vi "Initialize Central Message Handler.vi"(8 "Error In":errorcluster, 11 "Dashboard In":refnum<class "Dashboard.lvclass">) -> (0 "Error Out":errorcluster, 3 "Dashboard Out":refnum<class "Dashboard.lvclass">)   [LabVIEW 2019, in "Dashboard.lvclass"]
uses:
  Dashboard.lvclass
  Accessors/Processes/Get Processes.vi
  Process/Accessors/Message Queue/Get Message Queue.vi
  Accessors/Central Message Handler/Set Central Message Handler.vi
  Display Manager/Display Manager.lvclass
  Audio Analyzer/Audio Analyzer.lvclass
  Draw Frame/Draw Frame.lvclass
  Error Handling/Error Handling.lvclass
  Sequencer/Sequencer.lvclass
  Central Message Handler/Central Message Handler.lvclass
  Process/Process.lvclass
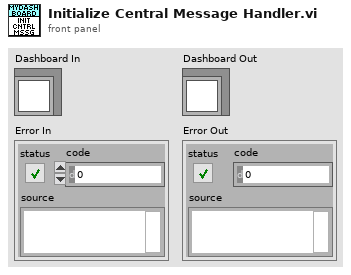
[diagram p1: front panel]
types:
  T1 = typedef "Dashboard.lvclass/Processes.ctl" = cluster{"Display Manager":refnum<class "Display Manager.lvclass">, "Audio Analyzer":refnum<class "Audio Analyzer.lvclass">, "Draw Frame":refnum<class "Draw Frame.lvclass">, "Error Handling":refnum<class "Error Handling.lvclass">, "Sequencer":refnum<class "Sequencer.lvclass">}
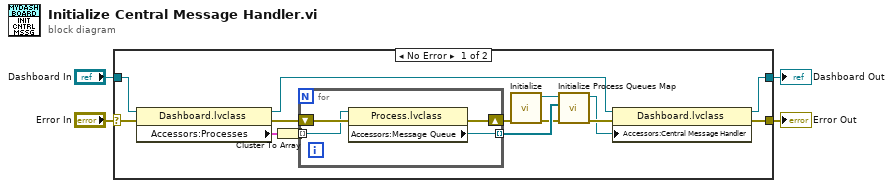
[diagram p0: block diagram]
diagram:
  n1 = case shown="No Error" "Error In" {
    selector: "Error In" -> [w16 w24]
    tunnel: [w18 w24] -> w4
    tunnel: [w17 w23] -> w3
    tunnel: "Dashboard In" -> [w15 w23]
    frame No Error {
      n2 = property class="Dashboard.lvclass"(reference=w15, error in=w16) -> (reference out=w14:refnum<class "Dashboard.lvclass">, error out=w11:errorcluster, "Accessors:Processes"=w13:T1)
      n3 = Cluster To Array(cluster=w13) -> (array=w12:refnum<class "Process.lvclass">[])
      n4 = for {
        tunnel: w12 -> [w21] mode=indexing
        shift-right: [w20] -> w10
        shift-left: w11 -> [w22]
        tunnel: [w19] -> w8 mode=indexing
        n5 = property class="Process.lvclass"(reference=w21, error in=w22) -> (error out=w20:errorcluster, "Accessors:Message Queue"=w19:refnum<queue>)  [unwired: 1 out]
      }
      n6 = call "Initialize.vi"("Error In"=w10) -> ("Error Out"=w7:errorcluster, "Central Message Handler"=w9:refnum<class "Central Message Handler.lvclass">)  [unwired: 9 in]
      n7 = call "Initialize Process Queues Map.vi"("Error In"=w7, "Processes Queues"=w8, "Central Message Handler In"=w9) -> ("Error Out"=w6:errorcluster, "Central Message Handler Out"=w5:refnum<class "Central Message Handler.lvclass">)  [unwired: 7 in]
      n8 = property class="Dashboard.lvclass"(reference=w14, error in=w6, "Accessors:Central Message Handler"=w5) -> (reference out=w17:refnum<class "Dashboard.lvclass">, error out=w18:errorcluster)
    }
    frame Error {
    }
  }
  "Error Out" <- w4
  "Dashboard Out" <- w3
